vi "Exercise1.22-Event-Blinking LED.vi"() -> ()   [LabVIEW 2013]
panel:
  in  "stop":bool
  out "LED Array":bool[](array[boolean])
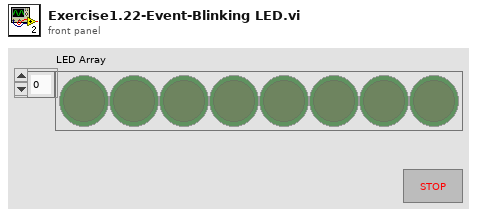
[diagram p1: front panel]
types:
  T1 = enum16{"State 0", "State 1", "State 2", "State 3", "State 4", "State 5", "State 6", "State 7", "State 8"}
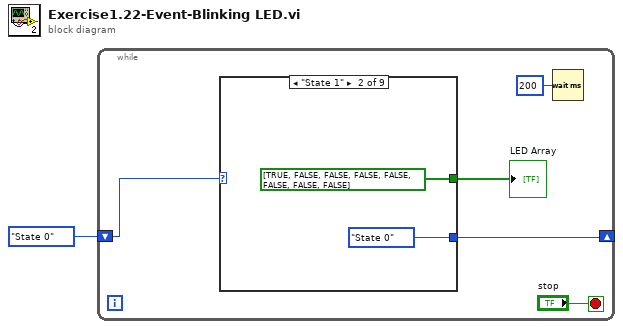
[diagram p0: block diagram]
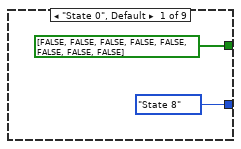
[diagram p2: hidden frame]
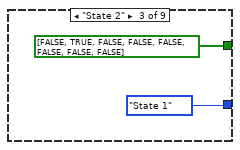
[diagram p3: hidden frame]
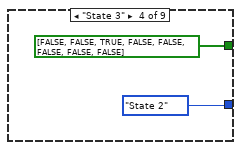
[diagram p4: hidden frame]
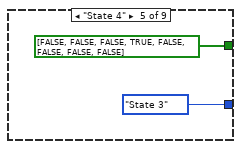
[diagram p5: hidden frame]
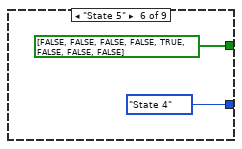
[diagram p6: hidden frame]
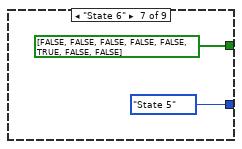
[diagram p7: hidden frame]
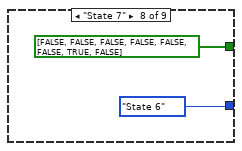
[diagram p8: hidden frame]
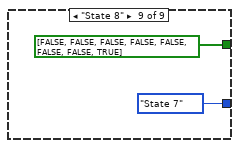
[diagram p9: hidden frame]
diagram:
  n1 = while {
    shift-right: [w3] -> _
    shift-left: T1."State 0" -> [w4]
    stop <- "stop" stop-if-true
    n2 = case shown="\"State 1\"" w4 {
      tunnel: [bool[] [FALSE, FALSE, FALSE, FALSE, FALSE, FALSE, FALSE, FALSE] bool[] [TRUE, FALSE, FALSE, FALSE, FALSE, FALSE, FALSE, FALSE] bool[] [FALSE, TRUE, FALSE, FALSE, FALSE, FALSE, FALSE, FALSE] bool[] [FALSE, FALSE, TRUE, FALSE, FALSE, FALSE, FALSE, FALSE] bool[] [FALSE, FALSE, FALSE, TRUE, FALSE, FALSE, FALSE, FALSE] bool[] [FALSE, FALSE, FALSE, FALSE, TRUE, FALSE, FALSE, FALSE] bool[] [FALSE, FALSE, FALSE, FALSE, FALSE, TRUE, FALSE, FALSE] bool[] [FALSE, FALSE, FALSE, FALSE, FALSE, FALSE, TRUE, FALSE] bool[] [FALSE, FALSE, FALSE, FALSE, FALSE, FALSE, FALSE, TRUE]] -> w6
      tunnel: [T1."State 8" T1."State 0" T1."State 1" T1."State 2" T1."State 3" T1."State 4" T1."State 5" T1."State 6" T1."State 7"] -> w3
      frame "State 0", Default {
      }
      frame "State 1" {
      }
      frame "State 2" {
      }
      frame "State 3" {
      }
      frame "State 4" {
      }
      frame "State 5" {
      }
      frame "State 6" {
      }
      frame "State 7" {
      }
      frame "State 8" {
      }
    }
    "LED Array" <- w6
    n3 = Wait (ms)(milliseconds to wait=u32 200) -> ()  [unwired: 1 out]
  }
